vi "MFLI worker -- V2.vi"(0 "PID parameters":T3={"P (sec)"=10.0, "I (sec)"=10.0}, 1 "MFLI controller action":T4=enum."Scan frequency", 5 "Address":string="DEV3523", 7 "lorentzian in":T1={"Amplitude"=0.013136296037631784, "omega(0)"=2004886.6969994097, "Gamma"=572.2011355500609, "phase"=4.6528430793035955, "Q"=3485.5434940490113, "Norm  Ampl"=nan, "z (inf)"=2.6950020505679743e-05+0.0007479581371481224i, "4corners"={"z (-pi/2)"=2.6670128459191578e-06+0.0007264075617308287i, "z(inf)"=2.6950020505679743e-05+0.0007479581371481224i, "z (pi/2)"=5.39944508838616e-06+0.0007722411448078829i, "z center"=4.033228967152659e-06+0.0007493243532693558i, "z(0)"=-1.8883562571374426e-05+0.0007506905693905893i, "radius"=2.295747984666925e-05}} {"z (inf)" format="%#9_9f"; "Q" format="%#9_9f"; "phase" format="%#9_9f"; "Gamma" format="%#9_9f"; "omega(0)" format="%#9_9f"}, 9 "sweep parameters":T5={"scan type"=enum."arctan", "N"=100, "cursor window"={"left"=32571.699125630872, "right "=32589.533031344432, "center"=32580.616078487652, "window"=17.83390571355876, "cursors"=[0, 1, 2], "relative"=0, "absolute"=0, "fixed vertical offset"=0.0, "vertical offset"=0.0, "skew"=0.0, "default window frac"=0.1, "kind"=enum."symmetric", "skew.left"=0.5, "skew.right"=0.5, "Plot ref"=refnum, "wing order"=enum."forw"}}, 11 "Error In":errorcluster, 12 "reqested size":i32=100, 13 "delay (msec)":i64=2) -> (6 "sweep time":dbl=1.133070214302279, 8 "lorentzian out":T1={"Amplitude"=0.013136296037631784, "omega(0)"=2004886.6969994097, "Gamma"=572.2011355500609, "phase"=4.6528430793035955, "Q"=3485.5434940490113, "Norm  Ampl"=nan, "z (inf)"=2.6950020505679743e-05+0.0007479581371481224i, "4corners"={"z (-pi/2)"=2.6670128459191578e-06+0.0007264075617308287i, "z(inf)"=2.6950020505679743e-05+0.0007479581371481224i, "z (pi/2)"=5.39944508838616e-06+0.0007722411448078829i, "z center"=4.033228967152659e-06+0.0007493243532693558i, "z(0)"=-1.8883562571374426e-05+0.0007506905693905893i, "radius"=2.295747984666925e-05}} {"z (inf)" format="%#9_9f"; "Q" format="%#9_9f"; "phase" format="%#9_9f"; "Gamma" format="%#9_9f"; "omega(0)" format="%#9_9f"}, 15 "Error Out":errorcluster)   [LabVIEW 2017]
uses:
  sweep parameters.ctl
  cursor winow.ctl
  MFLI controller action.ctl
  lorentzian.ctl
  circle corners.ctl
  pid -- parameters.ctl
  publisher action.ctl
  agregator -- action.ctl
  <instrlib>/Zurich Instruments LabOne/Zurich Instruments LabOne.lvlib
panel:
  out "scan progress":i32(slide) min=0 max=300 scale=0.0..300.0
  out "Thermometer":i32(slide) min=0 max=1 scale=0.0..100.0
  out "Selected Device":string="DEV3523"
  out "ind":i64=42
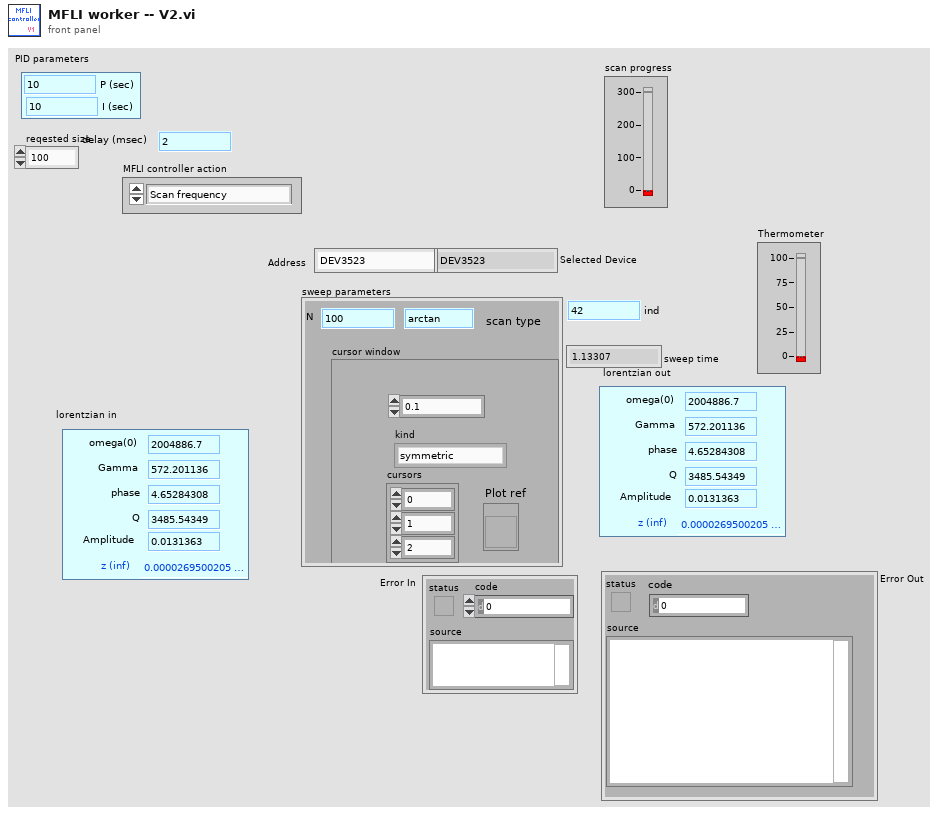
[diagram p1: front panel]
types:
  T1 = typedef "lorentzian.ctl" = cluster{"Amplitude":dbl, "omega(0)":dbl, "Gamma":dbl, "phase":dbl, "Q":dbl, "Norm  Ampl":dbl, "z (inf)":cdb, "4corners":T2}
  T2 = typedef "circle corners.ctl" = cluster{"z (-pi/2)":cdb, "z(inf)":cdb, "z (pi/2)":cdb, "z center":cdb, "z(0)":cdb, "radius":dbl}
  T3 = typedef "pid -- parameters.ctl" = cluster{"P (sec)":dbl, "I (sec)":dbl}
  T4 = typedef "MFLI controller action.ctl" = enum16{"Initialize", "Scan frequency", "open", "close", "read", "circle PLL"}
  T5 = typedef "sweep parameters.ctl" = cluster{"scan type":enum16{"linear", "arctan"}, "N":i64, "cursor window":T6}
  T6 = typedef "cursor winow.ctl" = cluster{"left":dbl, "right ":dbl, "center":dbl, "window":dbl, "cursors":i32[], "relative":i32, "absolute":i32, "fixed vertical offset":dbl, "vertical offset":dbl, "skew":dbl, "default window frac":dbl, "kind":enum16{"symmetric", "skewed", "fancy"}, "skew.left":dbl, "skew.right":dbl, "Plot ref":refnum<vi>, "wing order":enum16{"forw", "back"}}
  T7 = typedef "publisher action.ctl" = enum16{"set", "get"}
  T8 = typedef "agregator -- action.ctl" = enum16{"append", "interpolate", "empty!", "force", "init", "scale", "read last"}
  T9 = typedef "Zurich Instruments LabOne.lvlib/ziTypeHandle.ctl" = cluster{"handleValid":bool, "Conn":u64, "Path Prefix":string, "Handle":u64, "Connected":bool, "Clockbase(s)":dbl}
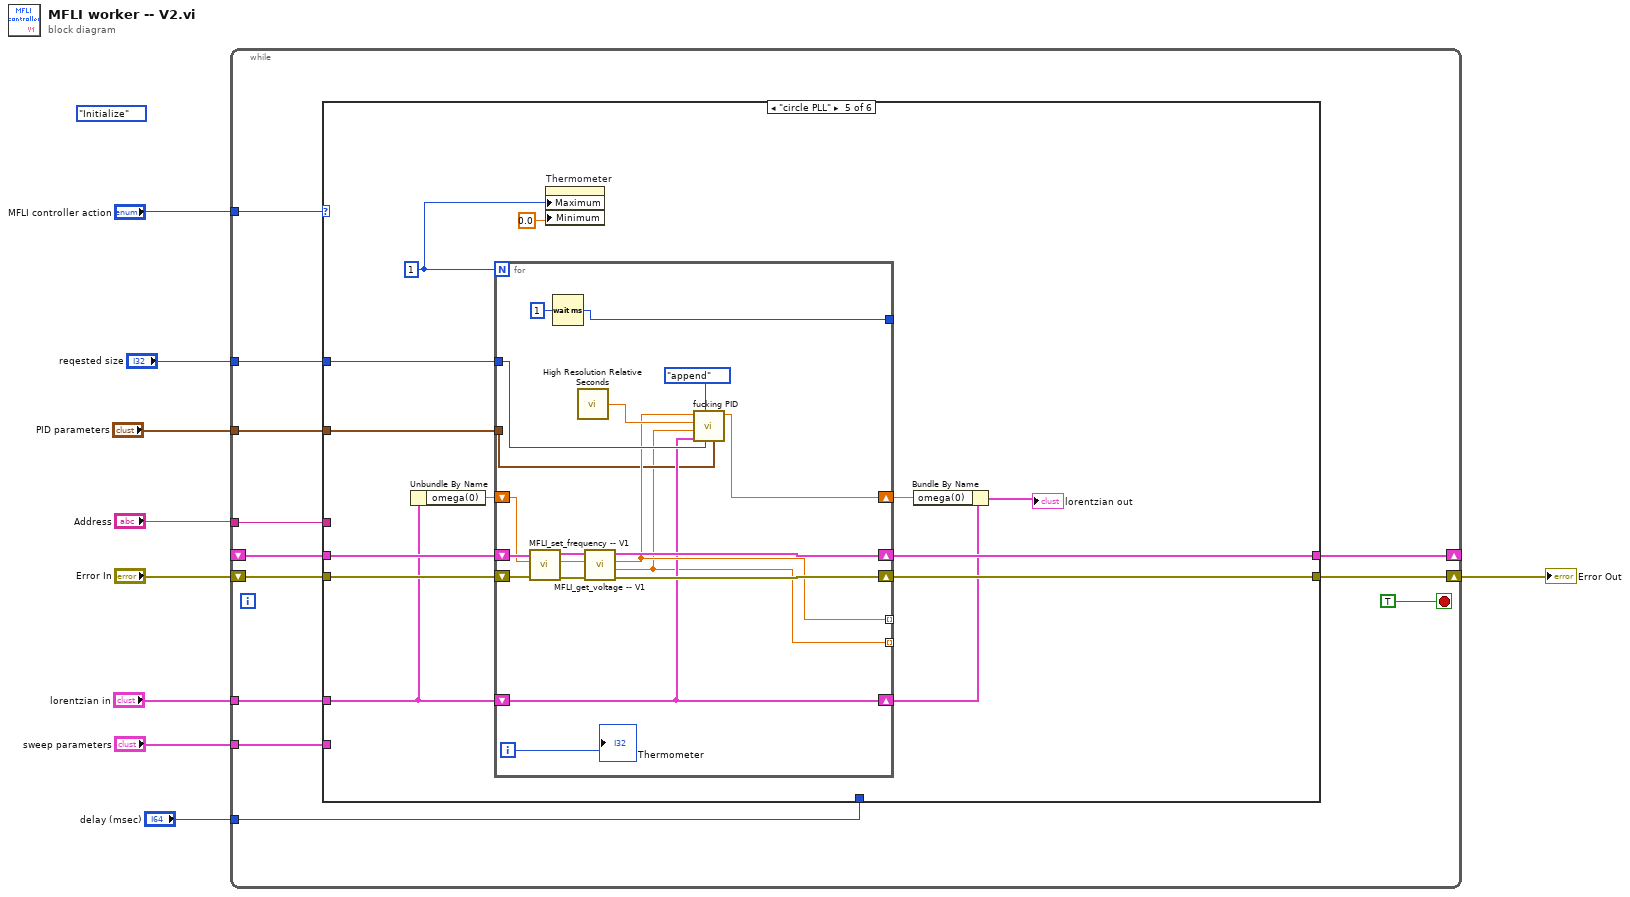
[diagram p0: block diagram]
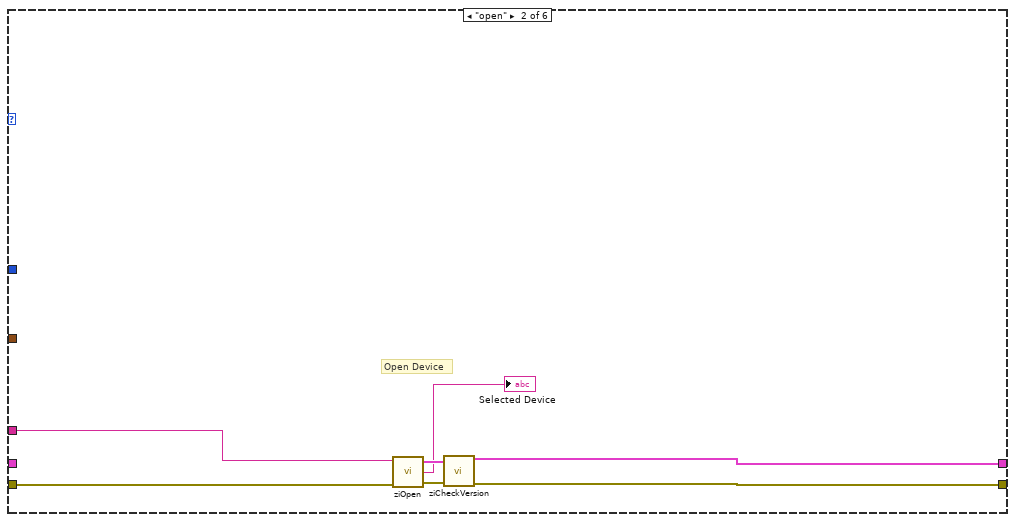
[diagram p3: hidden frame]
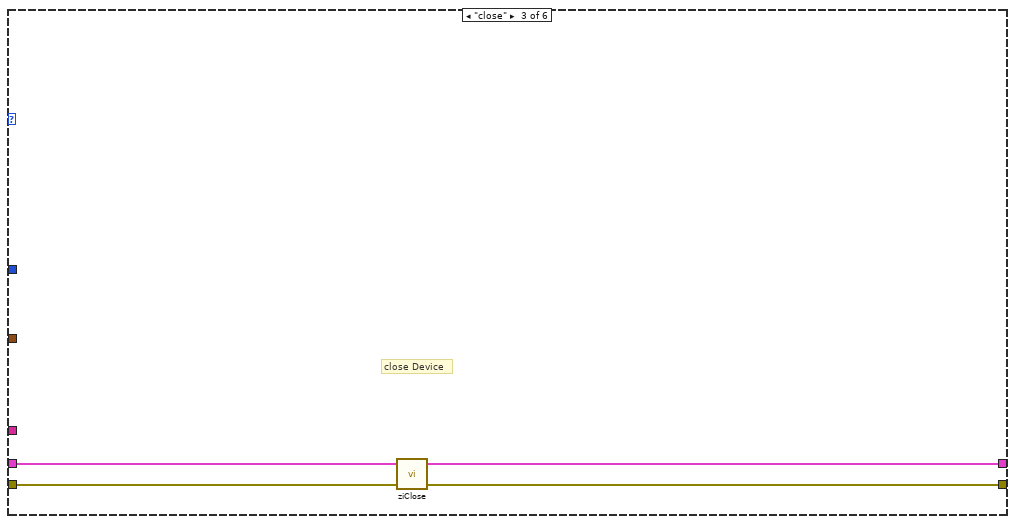
[diagram p4: hidden frame]
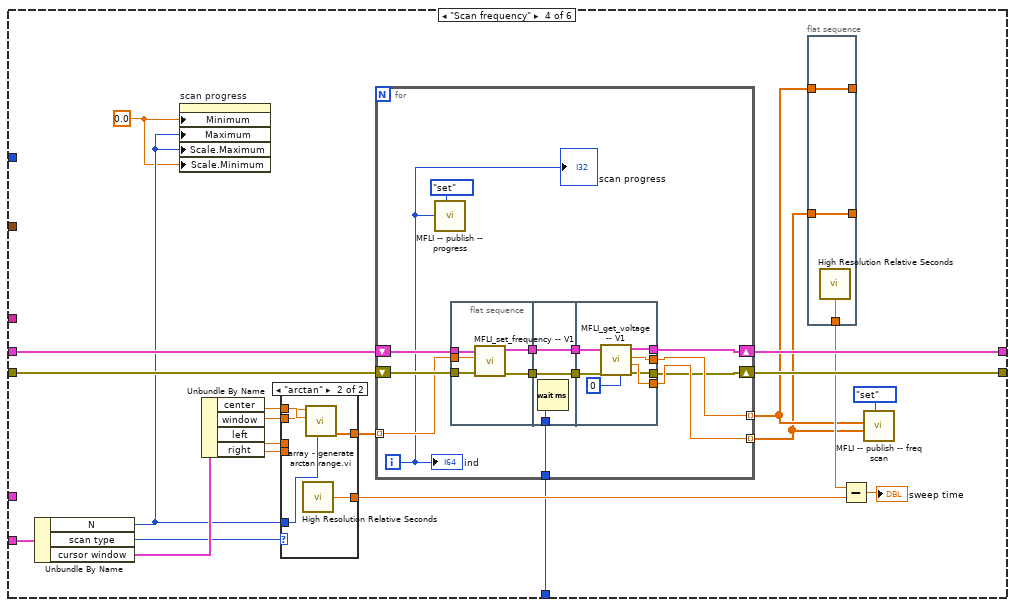
[diagram p5: hidden frame]
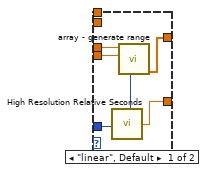
[diagram p6: hidden frame]
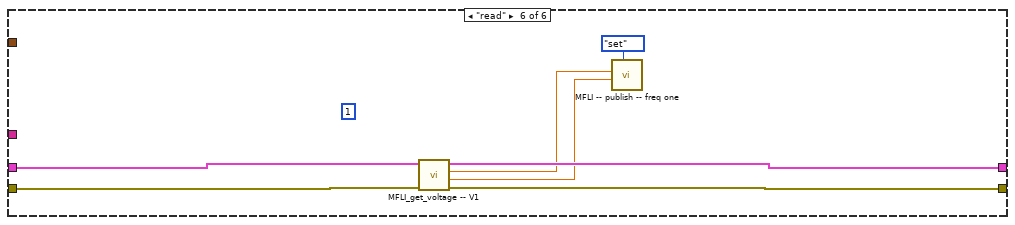
[diagram p7: hidden frame]
diagram:
  (unwired) MFLI_controller_action."Initialize" ("MFLI controller action")
  n1 = while {
    shift-right: [w19] -> _
    shift-left: _ -> [w20]
    shift-right: [w17] -> w5
    shift-left: "Error In" -> [w18]
    tunnel: "MFLI controller action" -> [w16]
    tunnel: "sweep parameters" -> [w15]
    tunnel: "Address" -> [w14]
    tunnel: "lorentzian in" -> [w13]
    tunnel: "PID parameters" -> [w12]
    tunnel: "reqested size" -> [w11]
    tunnel: "delay (msec)" -> [w10]
    stop <- TRUE stop-if-true
    n2 = case shown="\"circle PLL\"" w16 {
      tunnel: w20 -> [w23 _ w31 w54 w110 w136]
      tunnel: [w23 w24 w32 w53 w109 w135] -> w19
      tunnel: w18 -> [w22 w26 w34 w52 w108 w134]
      tunnel: [w22 w25 w33 w51 w107 w133] -> w17
      tunnel: w15 -> [_ _ _ w43 _ _]
      tunnel: w14 -> [_ w27 _ _ _ _]
      tunnel: w13 -> [_ _ _ _ w102 _]
      tunnel: w12 -> [_ _ _ _ w106 _]
      tunnel: w11 -> [_ _ _ _ w98 _]
      tunnel: w10 -> [_ _ _ w40 _ _]
      frame "Initialize", Default {
      }
      frame "open" {
        # "Open Device"
        n3 = call <instrlib>:"ziOpen.vi"("Error In"=w26, "Address"=w27) -> ("Error Out"=w30:errorcluster, "Selected Device"=→"Selected Device":string, "HandleOut"=w29:T9)  [unwired: 2 out]
        n4 = call <instrlib>:"ziCheckVersion.vi"("Handle In"=w29, "Error In"=w30) -> ("Handle Out"=w24:T9, "Error Out"=w25:errorcluster)  [unwired: 12 in]
      }
      frame "close" {
        # "close Device"
        n5 = call <instrlib>:"ziClose.vi"("Error In"=w34, "Handle In"=w31) -> ("Error Out"=w33:errorcluster, "Handle Out"=w32:T9)  [unwired: 2 in]
      }
      frame "Scan frequency" {
        w38 = 0.0 ("Data Entry Limits:Minimum")
        n6 = Unbundle By Name(w43) -> ("N"=w39:i64, "scan type"=w41:enum16{"linear", "arctan"}, "cursor window"=w42:T6)
        n7 = property on="scan progress" class="Slide (strict)"("Minimum"=w38, "Maximum"=w39, "Scale.Maximum"=w39, "Scale.Minimum"=w38) -> ()  [unwired: 2 in, 2 out]
        n8 = Unbundle By Name(w42) -> ("center"=w50:dbl, "window"=w49:dbl, "left"=w48:dbl, "right"=w47:dbl)
        n9 = case shown="\"arctan\"" w41 {
          tunnel: [w60 w65] -> w55
          tunnel: w50 -> [_ w64]
          tunnel: w49 -> [_ w63]
          tunnel: w48 -> [w59 _]
          tunnel: w47 -> [w58 _]
          tunnel: [w57 w62] -> w46
          tunnel: w39 -> [w56 w61]
          frame "linear", Default {
            n10 = call <vilib>:"High Resolution Relative Seconds.vi"() -> ("relative seconds"=w57:dbl)
            n11 = call "array - generate range.vi"("N"=w56, "freq max"=w58, "freq min"=w59) -> ("Array"=w60:dbl[])  [unwired: 7 in, 1 out]
          }
          frame "arctan" {
            n12 = call <vilib>:"High Resolution Relative Seconds.vi"() -> ("relative seconds"=w62:dbl)
            n13 = call "array - generate arctan range.vi.vi"("N"=w61, "omega0"=w64, "gamma"=w63) -> ("Array"=w65:dbl[])  [unwired: 8 in]
          }
        }
        n14 = for {
          shift-right: [w69] -> w53
          shift-left: w54 -> [w79]
          shift-right: [w68] -> w51
          shift-left: w52 -> [w78]
          tunnel: w55 -> [w77] mode=indexing
          tunnel: [w71] -> w37 mode=indexing
          tunnel: [w70] -> w36 mode=indexing
          tunnel: w40 -> [w72]
          i -> [w66]
          n15 = call "MFLI -- publish -- progress.vi"("publisher action"=publisher_action."set", "num"=w66) -> ()  [unwired: 9 in, 1 out]
          n16 = flat-sequence {
            tunnel: w79 -> [w84]
            tunnel: w78 -> [w82]
            tunnel: w77 -> [w80]
            tunnel: [w83] -> w76
            tunnel: [w81] -> w75
            tunnel: w76 -> [w85]
            tunnel: w75 -> [w87]
            tunnel: [w85] -> w74
            tunnel: [w87] -> w73
            tunnel: w72 -> [w86]
            tunnel: [w88] -> w68
            tunnel: w74 -> [w91]
            tunnel: w73 -> [w89]
            tunnel: [w94] -> w71
            tunnel: [w93] -> w70
            tunnel: [w90] -> w69
            frame #0 {
              n17 = call "MFLI_set_frequency -- V1.vi"("Error In"=w82, "Freq in (Hz)"=w80, "Handle In"=w84) -> ("Error Out"=w81:errorcluster, "Handle Out"=w83:T9)  [unwired: 5 in, 2 out]
            }
            frame #1 {
              n18 = Wait (ms)(milliseconds to wait=w86) -> ()  [unwired: 1 out]
            }
            frame #2 {
              n19 = call "MFLI_get_voltage -- V1.vi"("Oscillator (0)"=u16 0, "Error In"=w89, "Handle In"=w91) -> ("Error Out"=w88:errorcluster, "z out (V)"=w93:cdb, "Freq out (Hz)"=w94:dbl, "Handle Out"=w90:T9)  [unwired: 5 in]
            }
          }
          "ind" <- w66
          "scan progress" <- w66
        }
        n20 = flat-sequence {
          tunnel: w37 -> [w97]
          tunnel: [w97] -> _
          tunnel: w36 -> [w96]
          tunnel: [w96] -> _
          tunnel: [w95] -> w45
          frame #0 {
            n21 = call <vilib>:"High Resolution Relative Seconds.vi"() -> ("relative seconds"=w95:dbl)
          }
        }
        n22 = Subtract(x=w45, y=w46) -> (x-y=→"sweep time":dbl)
        n23 = call "MFLI -- publish -- freq scan.vi"("publisher action"=publisher_action."set", "Voltage IN (V)"=w36, "Freq IN (Hz)"=w37) -> ()  [unwired: 7 in, 2 out]
      }
      frame "circle PLL" {
        w103 = 1
        n24 = Unbundle By Name(w102) -> ("omega(0)"=w104:dbl)
        n25 = for {
          N: w103 -> [_]
          shift-right: [w128] -> w109
          shift-left: w110 -> [w127]
          shift-right: [w129] -> w107
          shift-left: w108 -> [w125]
          tunnel: [w117] -> _ mode=indexing
          tunnel: [w111] -> _ mode=indexing
          tunnel: w98 -> [w118]
          shift-right: [w114] -> w101
          shift-left: w104 -> [w116]
          tunnel: w106 -> [w112]
          tunnel: [w115] -> _
          shift-right: [w113] -> w99
          shift-left: w102 -> [w113]
          i -> [w123]
          n26 = call "MFLI_set_frequency -- V1.vi"("Error In"=w125, "Freq in (Hz)"=w116, "Handle In"=w127) -> ("Error Out"=w124:errorcluster, "Freq out (Hz)"=w121:dbl, "Handle Out"=w126:T9)  [unwired: 5 in, 1 out]
          n27 = Wait (ms)(milliseconds to wait=u32 1) -> (millisecond timer value=w115:u32)
          n28 = call <vilib>:"High Resolution Relative Seconds.vi"() -> ("relative seconds"=w120:dbl)
          n29 = call "MFLI_get_voltage -- V1.vi"("Error In"=w124, "Freq IN (Hz)"=w121, "Handle In"=w126) -> ("Error Out"=w129:errorcluster, "z out (V)"=w111:cdb, "Freq out (Hz)"=w117:dbl, "Handle Out"=w128:T9)  [unwired: 5 in]
          n30 = call "fucking PID.vi"("PID parameters"=w112, "requested size"=w118, "PID action"=agregator_--_action."append", "lorentzian IN"=w113, "voltage IN (V)"=w111, "time in (sec)"=w120, "frequency IN (Hz)"=w117) -> ("frequency out (Hz)"=w114:dbl)  [unwired: 1 in, 3 out]
          "Thermometer" <- w123
        }
        n31 = property on="Thermometer" class="Slide (strict)"("Maximum"=w103, "Minimum"=0.0 ("Data Entry Limits:Minimum")) -> ()  [unwired: 2 in, 2 out]
        n32 = Bundle By Name(cluster=w99, "omega(0)"=w101) -> (→"lorentzian out":T1)
      }
      frame "read" {
        (unwired) 1
        n33 = call "MFLI_get_voltage -- V1.vi"("Error In"=w134, "Handle In"=w136) -> ("Error Out"=w133:errorcluster, "z out (V)"=w131:cdb, "Freq out (Hz)"=w132:dbl, "Handle Out"=w135:T9)  [unwired: 6 in]
        n34 = call "MFLI -- publish -- freq one.vi"("publisher action"=publisher_action."set", "Voltage IN (V)"=w131, "freq IN (Hz)"=w132) -> ()  [unwired: 7 in, 2 out]
      }
    }
  }
  "Error Out" <- w5
